vi "Test Basic Function 2.vi"() -> ()   [LabVIEW 2014]
uses:
  <vilib>/Aledyne-TSXperts/Arduino Compatible Compiler for LabVIEW/addons/Arduino Math/Arduino Math.lvlib
panel:
  out "result 5":sgl
  out "result 4":sgl
  out "result 3":sgl
  out "result 2":sgl
  out "result":sgl
  out "Error Out":errorcluster
  in  "Error In":errorcluster
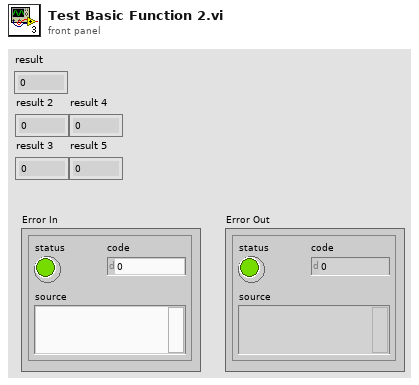
[diagram p1: front panel]
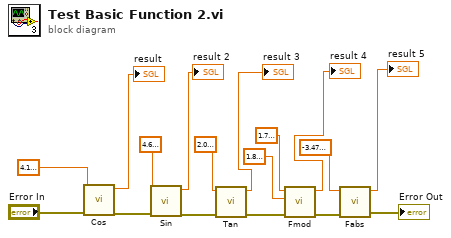
[diagram p0: block diagram]
diagram:
  n1 = call <vilib>:"Cos.vi"("Error In"="Error In", "x"=sgl 4.2) -> ("Error Out"=w10:errorcluster, "result"=→"result":sgl)  [unwired: 8 in]
  n2 = call <vilib>:"Sin.vi"("Error In"=w10, "x"=sgl 4.7) -> ("Error Out"=w11:errorcluster, "sin(x)"=→"result 2":sgl)  [unwired: 8 in]
  n3 = call <vilib>:"Tan.vi"("Error In"=w11, "x"=sgl 2.1) -> ("Error Out"=w12:errorcluster, "tan(x)"=→"result 3":sgl)  [unwired: 8 in]
  n4 = call <vilib>:"Fmod.vi"("Error In"=w12, "y"=sgl 1.9 ("x"), "x"=sgl 1.8) -> ("Error Out"=w13:errorcluster, "fmod(x,y)"=→"result 4":sgl)  [unwired: 7 in]
  n5 = call <vilib>:"Fabs.vi"("Error In"=w13, "x"=sgl -3.47) -> ("Error Out"=→"Error Out":errorcluster, "result"=→"result 5":sgl)  [unwired: 8 in]
